vi "QAM Symbol to Bitstream.vi"(1 "Symbol In":cdb[](array[numeric]), 2 "QAM Complexity":T1(ring)) -> (0 "BitStream Out":i32[](array[numeric]))   [LabVIEW 2018]
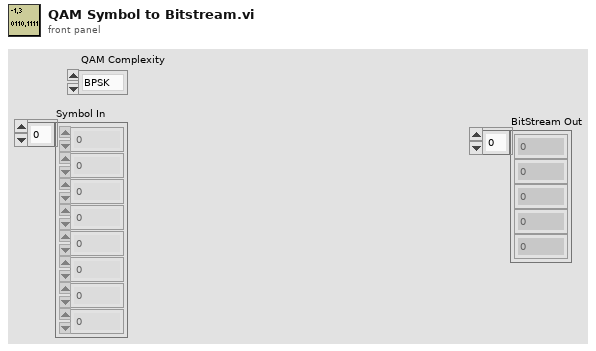
[diagram p1: front panel]
types:
  T1 = enum16{"BPSK", "QPSK", "16-QAM", "64-QAM", "256-QAM"}
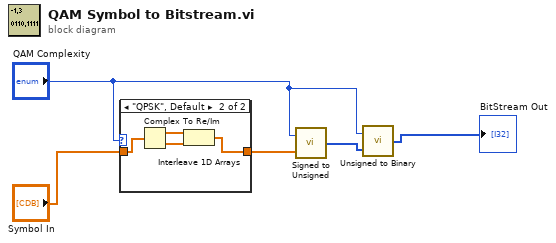
[diagram p0: block diagram]
diagram:
  n1 = case shown="\"QPSK\", Default" "QAM Complexity" {
    tunnel: "Symbol In" -> [w6 w8]
    tunnel: [w6 w7] -> w4
    frame "BPSK" {
    }
    frame "QPSK", Default {
      n2 = Complex To Re/Im(x + iy=w8) -> (x=w10:dbl[], y=w9:dbl[])
      n3 = Interleave 1D Arrays(w10, w9) -> (w7:dbl[])
    }
  }
  n4 = call "Signed to Unsigned.vi"("Symbol In"=w4, "QAM Complexity"="QAM Complexity") -> ("BitStream Out"=w2:i32[])
  n5 = call "Unsigned to Binary.vi"("UInt In"=w2, "QAM Complexity"="QAM Complexity") -> ("BitStream Out"=→"BitStream Out":i32[])
